vi "generateDecimalFractions.vi"(6 "timeout (10000)":i32=10000, 8 "error in (no error)":errorcluster, 11 "Parameters":T2={"params"={"apiKey"="", "n"=0, "decimalPlaces"=0, "replacement"=TRUE}, "id"=0.0}) -> (0 "error out":errorcluster, 3 "Response":T1 {"result"."random"."data" format="%#_14g"}, 4 "error data":string[](array[string]))   [LabVIEW 2014, in "Random JSON API.lvlib"]
uses:
  Random JSON API.lvlib
  Type Defs/generateDecimalFractionsRequest.ctl
  Type Defs/generateDecimalFractionsResponse.ctl
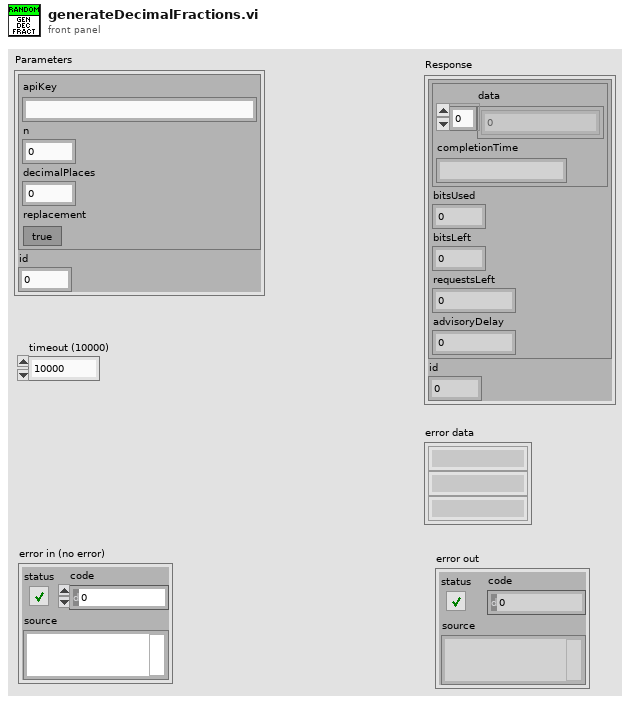
[diagram p1: front panel]
types:
  T1 = typedef "Random JSON API.lvlib/generateDecimalFractionsResponse.ctl" = cluster{"result":cluster{"random":cluster{"data":dbl[], "completionTime":string}, "bitsUsed":i32, "bitsLeft":i32, "requestsLeft":i32, "advisoryDelay":i32}, "id":dbl}
  T2 = typedef "Random JSON API.lvlib/generateDecimalFractionsRequest.ctl" = cluster{"params":cluster{"apiKey":string, "n":i32, "decimalPlaces":i32, "replacement":bool}, "id":dbl}
  T3 = cluster{"apiKey":string, "n":i32, "decimalPlaces":i32, "replacement":bool}
  T4 = cluster{"jsonrpc":string, "method":string, "params":cluster{"apiKey":string, "n":i32, "decimalPlaces":i32, "replacement":bool}, "id":dbl}
  T5 = cluster{"completionTime":string, "bitsUsed":i32, "bitsLeft":i32, "requestsLeft":i32, "advisoryDelay":i32}
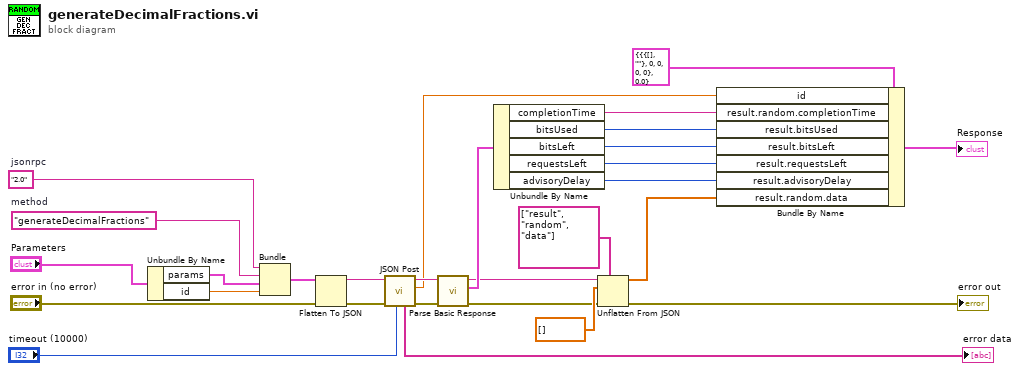
[diagram p0: block diagram]
diagram:
  w14 = "2.0"  # jsonrpc
  w18 = "generateDecimalFractions"  # method
  n1 = Unbundle By Name("Parameters") -> ("params"=w17:T3, "id"=w16:dbl)
  n2 = Bundle("jsonrpc"=w14, "method"=w18, "params"=w17, "id"=w16) -> (w15:T4)  [unwired: 1 in]
  n3 = Flatten To JSON(anything=w15, error in (no error)="error in (no error)") -> (JSON string=w20:string, 11:w21:errorcluster)  [unwired: 1 in]
  n4 = call "JSON Post.vi"("timeout (10000)"="timeout (10000)", "error in (no error)"=w21, "Request JSON String"=w20) -> ("error out"=w27:errorcluster, "id"=w10:dbl, "Response JSON String"=w11:string, "error data"=→"error data":string[])  [unwired: 5 in]
  n5 = call "Parse Basic Response.vi"("error in (no error)"=w27, "body in"=w11) -> ("error out"=w8:errorcluster, "result cluster"=w9:T5, "body out"=w5:string)  [unwired: 7 in]
  n6 = Unbundle By Name(w9) -> ("completionTime"=w26:string, "bitsUsed"=w25:i32, "bitsLeft"=w24:i32, "requestsLeft"=w23:i32, "advisoryDelay"=w22:i32)
  n7 = Unflatten From JSON(path=string[] ["result", "random", "data"], JSON string=w5, type and defaults=dbl[] [], error in (no error)=w8) -> (value=w6:dbl[], error out=→"error out":errorcluster)  [unwired: 3 in]
  n8 = Bundle By Name(cluster=T1 {"result"={"random"={"data"=[], "completionTime"=""}, "bitsUsed"=0, "bitsLeft"=0, "requestsLeft"=0, "advisoryDelay"=0}, "id"=0.0} ("Response"), "id"=w10, "result.random.completionTime"=w26, "result.bitsUsed"=w25, "result.bitsLeft"=w24, "result.requestsLeft"=w23, "result.advisoryDelay"=w22, "result.random.data"=w6) -> (→"Response":T1)
